vi "SetParameterVariantToData.vi"(8 "error in":errorcluster, 10 "Command":string, 11 "Parameters":string[](array[string])) -> (0 "error out":errorcluster, 3 "SetParameterInputs":T1)   [LabVIEW 2018, in "AcPwrPlugins.lvlib" / "AcPwrBase.lvclass"]
uses:
  AcPwrBase.lvclass
  TypeDefs/SetParameterInputs.ctl
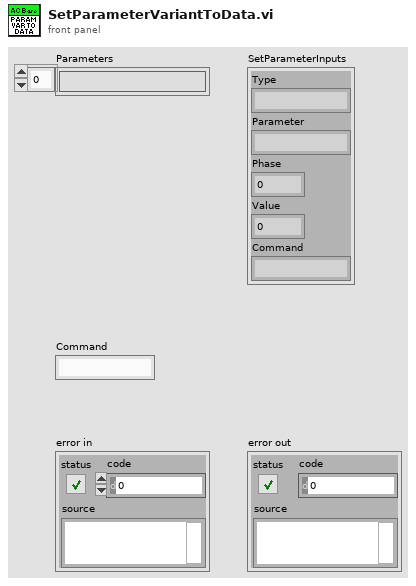
[diagram p1: front panel]
types:
  T1 = typedef "AcPwrPlugins.lvlib/AcPwrBase.lvclass/SetParameterInputs.ctl" = cluster{"Type":string, "Parameter":string, "Phase":i32, "Value":dbl, "Command":string}
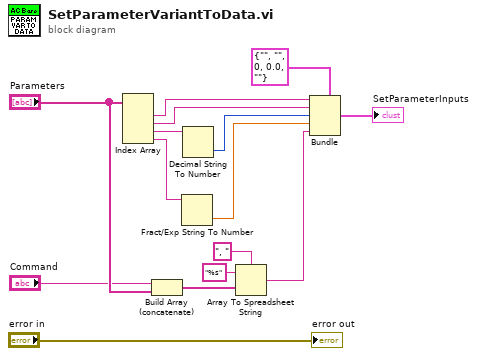
[diagram p0: block diagram]
diagram:
  n1 = Index Array(array="Parameters") -> (element #1=w10:string, element #2=w9:string, element #3=w14:string, element #4=w15:string)  [unwired: 4 in]
  n2 = Build Array (concatenate)("Command", "Parameters") -> (w3:string[])
  n3 = Fract/Exp String To Number(string=w15) -> (number=w7:dbl)  [unwired: 3 in, 1 out]
  n4 = Decimal String To Number(string=w14) -> (number=w8:i32)  [unwired: 2 in, 1 out]
  n5 = Array To Spreadsheet String(delimiter (Tab)=", ", array=w3, 3:"%s" ("format string")) -> (spreadsheet string=w1:string)
  n6 = Bundle(cluster=T1 {"Type"="", "Parameter"="", "Phase"=0, "Value"=0.0, "Command"=""} ("SetParameterInputs"), "Type"=w10, "Parameter"=w9, "Phase"=w8, "Value"=w7, "Command"=w1) -> (→"SetParameterInputs":T1)
  "error out" <- "error in"
